vi "XIPIN_SMPTE2022-5_6_Video_over_IP_Transmitter_2_1.vi"   [LabVIEW 2017]
doc: "The Xilinx LogiCORE IP SMPTE2022-5/6 Video over IP Transmitter is a module for broadcast applications that requires bridging between SMPTE video connectivity standards (SD/HD/ 3G-SDI) and 10 Gb/s networks. It is capable of mapping SD/HD/3G-SDI video streams into Ethernet packets and adding systematically generated redundant data.\n------------------------------------\n<b>Need License</b> : Yes\n<b>Interface</b> : AXI4 AXI4-Stream AXI4-Lite"
uses:
  <vilib>/rvi/XilinxIP/XIPIN_XNode/niFpgaXIPIN.xnode
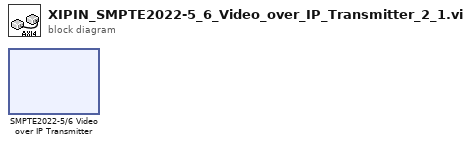
[diagram p0: block diagram]
diagram:
  n1 = xnode ("SMPTE2022-5/6 Video over IP Transmitter")() -> ()
